vi "RT 4Servos Module.vi"(0 "FPGA VI Reference In":refnum<k20>, 1 "Angle 1":u32=130, 2 "Angle 2":u32=130, 3 "Angle 3":u32=130, 4 "Angle 4":u32=130, 5 "Error In":errorcluster, 6 "Motor 1":enum32{"B", "S", "E", "C"}(ring), 7 "Arm":enum32{"meArm", "uArm"}(ring), 8 "Motor 2":enum32{"B", "S", "E", "C"}(ring)=enum."S", 10 "Motor 3":enum32{"B", "S", "E", "C"}(ring)=enum."E", 11 "No. of Motors":enum32{"1", "2", "3", "4"}(ring), 12 "Motor 4":enum32{"B", "S", "E", "C"}(ring)=enum."C") -> (14 "FPGA VI Reference Out":refnum<k20>, 19 "Error Out":errorcluster)   [LabVIEW 2015]
uses:
  <vilib>/Utility/error.llb/Error Cluster From Error Code.vi
  <vilib>/rvi/errors/niLvFpgaAdjustHostInterfaceError.vi
  <vilib>/rvi/interface/nirviReadWriteControl/nirviReadWriteControl.xnode
  NiFpgaLv.dll
  <vilib>/rvi/interface/Simulation/niFpgaSimulationCallBeginRW.vi
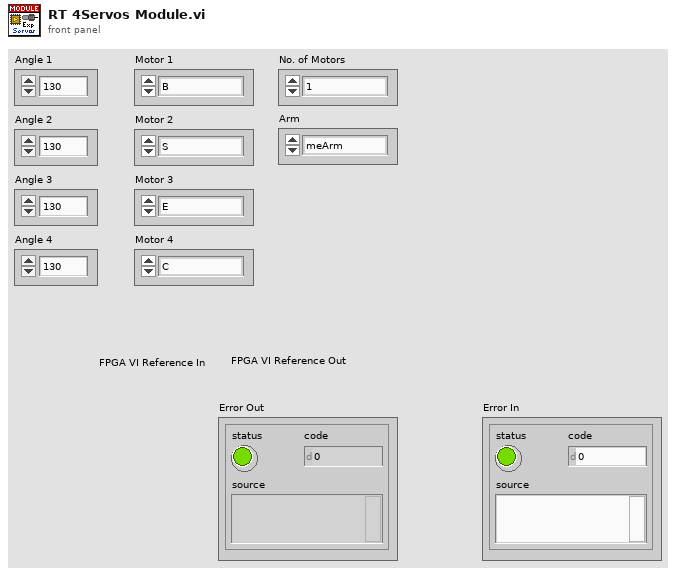
[diagram p1: front panel]
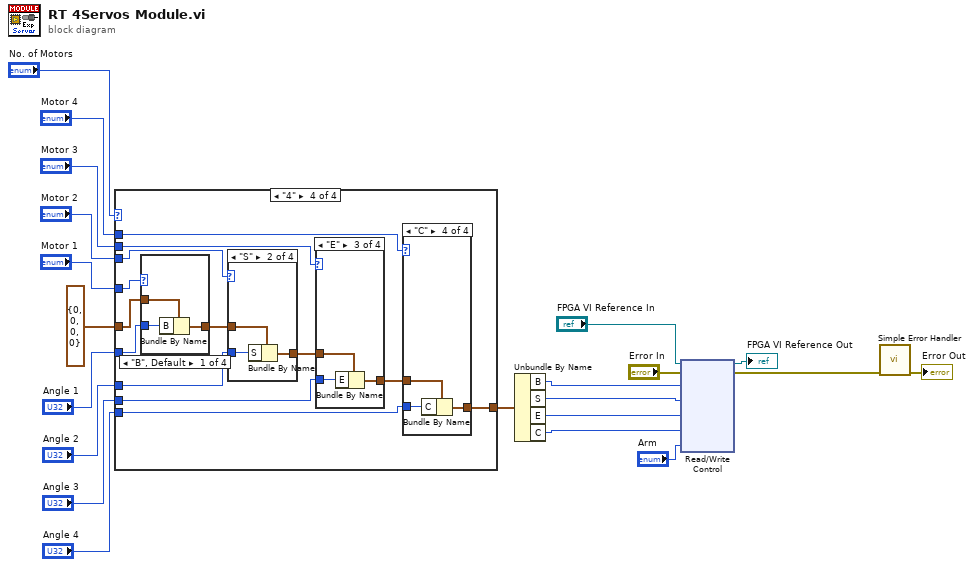
[diagram p0: block diagram]
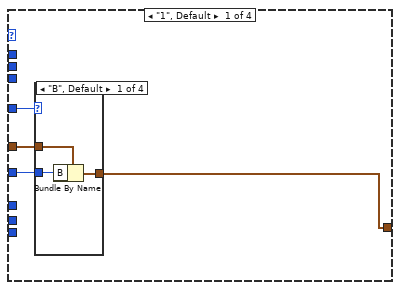
[diagram p2: hidden frame]
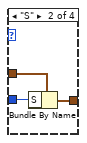
[diagram p3: hidden frame]
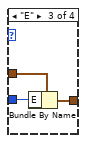
[diagram p4: hidden frame]
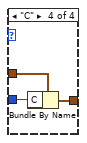
[diagram p5: hidden frame]
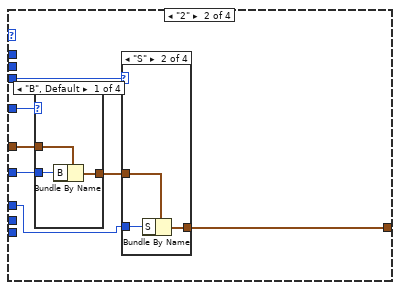
[diagram p6: hidden frame]
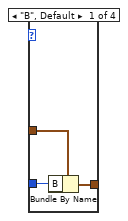
[diagram p7: hidden frame]
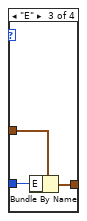
[diagram p8: hidden frame]
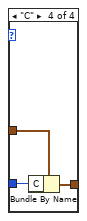
[diagram p9: hidden frame]
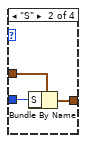
[diagram p10: hidden frame]
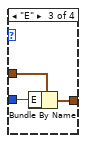
[diagram p11: hidden frame]
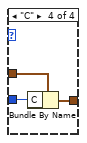
[diagram p12: hidden frame]
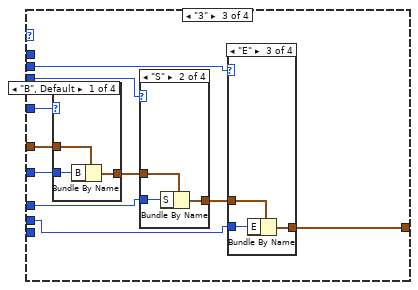
[diagram p13: hidden frame]
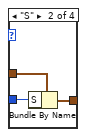
[diagram p14: hidden frame]
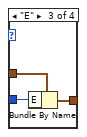
[diagram p15: hidden frame]
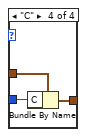
[diagram p16: hidden frame]
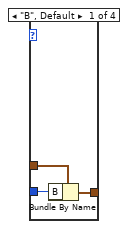
[diagram p17: hidden frame]
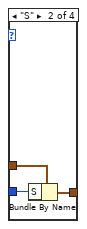
[diagram p18: hidden frame]
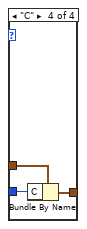
[diagram p19: hidden frame]
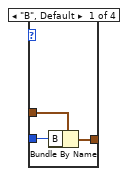
[diagram p20: hidden frame]
diagram:
  n1 = case shown="\"4\"" "No. of Motors" {
    tunnel: "Motor 1" -> [w25 w39 w74 w122]
    tunnel: "Motor 3" -> [_ _ w69 w120]
    tunnel: "Motor 4" -> [_ _ _ w119]
    tunnel: "Motor 2" -> [_ w38 w73 w121]
    tunnel: "Angle 4" -> [_ _ _ w115]
    tunnel: "Angle 2" -> [_ w41 w71 w117]
    tunnel: "Angle 3" -> [_ _ w70 w116]
    tunnel: "Angle 1" -> [w23 w42 w72 w118]
    tunnel: cluster{"B":u32, "S":u32, "E":u32, "C":u32} {"B"=0, "S"=0, "E"=0, "C"=0} ("Servos") -> [w24 w44 w76 w123]
    tunnel: [w22 w43 w77 w124] -> w10
    frame "1", Default {
      n2 = case shown="\"B\", Default" w25 {
        tunnel: w24 -> [w28 w31 w34 w36]
        tunnel: w23 -> [w26 w30 w32 w35]
        tunnel: [w27 w29 w33 w37] -> w22
        frame "B", Default {
          n3 = Bundle By Name(cluster=w28, "B"=w26) -> (w27:cluster{"B":u32, "S":u32, "E":u32, "C":u32})
        }
        frame "S" {
          n4 = Bundle By Name(cluster=w31, "S"=w30) -> (w29:cluster{"B":u32, "S":u32, "E":u32, "C":u32})
        }
        frame "E" {
          n5 = Bundle By Name(cluster=w34, "E"=w32) -> (w33:cluster{"B":u32, "S":u32, "E":u32, "C":u32})
        }
        frame "C" {
          n6 = Bundle By Name(cluster=w36, "C"=w35) -> (w37:cluster{"B":u32, "S":u32, "E":u32, "C":u32})
        }
      }
    }
    frame "2" {
      n7 = case shown="\"B\", Default" w39 {
        tunnel: w44 -> [w59 w62 w65 w68]
        tunnel: w42 -> [w57 w61 w63 w67]
        tunnel: [w58 w60 w64 w66] -> w40
        frame "B", Default {
          n8 = Bundle By Name(cluster=w59, "B"=w57) -> (w58:cluster{"B":u32, "S":u32, "E":u32, "C":u32})
        }
        frame "S" {
          n9 = Bundle By Name(cluster=w62, "S"=w61) -> (w60:cluster{"B":u32, "S":u32, "E":u32, "C":u32})
        }
        frame "E" {
          n10 = Bundle By Name(cluster=w65, "E"=w63) -> (w64:cluster{"B":u32, "S":u32, "E":u32, "C":u32})
        }
        frame "C" {
          n11 = Bundle By Name(cluster=w68, "C"=w67) -> (w66:cluster{"B":u32, "S":u32, "E":u32, "C":u32})
        }
      }
      n12 = case shown="\"S\"" w38 {
        tunnel: w40 -> [w47 w50 w53 w55]
        tunnel: w41 -> [w45 w49 w51 w54]
        tunnel: [w46 w48 w52 w56] -> w43
        frame "B", Default {
          n13 = Bundle By Name(cluster=w47, "B"=w45) -> (w46:cluster{"B":u32, "S":u32, "E":u32, "C":u32})
        }
        frame "S" {
          n14 = Bundle By Name(cluster=w50, "S"=w49) -> (w48:cluster{"B":u32, "S":u32, "E":u32, "C":u32})
        }
        frame "E" {
          n15 = Bundle By Name(cluster=w53, "E"=w51) -> (w52:cluster{"B":u32, "S":u32, "E":u32, "C":u32})
        }
        frame "C" {
          n16 = Bundle By Name(cluster=w55, "C"=w54) -> (w56:cluster{"B":u32, "S":u32, "E":u32, "C":u32})
        }
      }
    }
    frame "3" {
      n17 = case shown="\"B\", Default" w74 {
        tunnel: w76 -> [w81 w84 w87 w90]
        tunnel: w72 -> [w79 w83 w85 w89]
        tunnel: [w80 w82 w86 w88] -> w75
        frame "B", Default {
          n18 = Bundle By Name(cluster=w81, "B"=w79) -> (w80:cluster{"B":u32, "S":u32, "E":u32, "C":u32})
        }
        frame "S" {
          n19 = Bundle By Name(cluster=w84, "S"=w83) -> (w82:cluster{"B":u32, "S":u32, "E":u32, "C":u32})
        }
        frame "E" {
          n20 = Bundle By Name(cluster=w87, "E"=w85) -> (w86:cluster{"B":u32, "S":u32, "E":u32, "C":u32})
        }
        frame "C" {
          n21 = Bundle By Name(cluster=w90, "C"=w89) -> (w88:cluster{"B":u32, "S":u32, "E":u32, "C":u32})
        }
      }
      n22 = case shown="\"S\"" w73 {
        tunnel: w75 -> [w105 w108 w111 w113]
        tunnel: w71 -> [w103 w107 w109 w112]
        tunnel: [w104 w106 w110 w114] -> w78
        frame "B", Default {
          n23 = Bundle By Name(cluster=w105, "B"=w103) -> (w104:cluster{"B":u32, "S":u32, "E":u32, "C":u32})
        }
        frame "S" {
          n24 = Bundle By Name(cluster=w108, "S"=w107) -> (w106:cluster{"B":u32, "S":u32, "E":u32, "C":u32})
        }
        frame "E" {
          n25 = Bundle By Name(cluster=w111, "E"=w109) -> (w110:cluster{"B":u32, "S":u32, "E":u32, "C":u32})
        }
        frame "C" {
          n26 = Bundle By Name(cluster=w113, "C"=w112) -> (w114:cluster{"B":u32, "S":u32, "E":u32, "C":u32})
        }
      }
      n27 = case shown="\"E\"" w69 {
        tunnel: w78 -> [w93 w96 w99 w101]
        tunnel: [w92 w95 w98 w102] -> w77
        tunnel: w70 -> [w91 w94 w97 w100]
        frame "B", Default {
          n28 = Bundle By Name(cluster=w93, "B"=w91) -> (w92:cluster{"B":u32, "S":u32, "E":u32, "C":u32})
        }
        frame "S" {
          n29 = Bundle By Name(cluster=w96, "S"=w94) -> (w95:cluster{"B":u32, "S":u32, "E":u32, "C":u32})
        }
        frame "E" {
          n30 = Bundle By Name(cluster=w99, "E"=w97) -> (w98:cluster{"B":u32, "S":u32, "E":u32, "C":u32})
        }
        frame "C" {
          n31 = Bundle By Name(cluster=w101, "C"=w100) -> (w102:cluster{"B":u32, "S":u32, "E":u32, "C":u32})
        }
      }
    }
    frame "4" {
      n32 = case shown="\"B\", Default" w122 {
        tunnel: w123 -> [w130 w133 w136 w138]
        tunnel: w118 -> [w128 w132 w134 w137]
        tunnel: [w129 w131 w135 w139] -> w127
        frame "B", Default {
          n33 = Bundle By Name(cluster=w130, "B"=w128) -> (w129:cluster{"B":u32, "S":u32, "E":u32, "C":u32})
        }
        frame "S" {
          n34 = Bundle By Name(cluster=w133, "S"=w132) -> (w131:cluster{"B":u32, "S":u32, "E":u32, "C":u32})
        }
        frame "E" {
          n35 = Bundle By Name(cluster=w136, "E"=w134) -> (w135:cluster{"B":u32, "S":u32, "E":u32, "C":u32})
        }
        frame "C" {
          n36 = Bundle By Name(cluster=w138, "C"=w137) -> (w139:cluster{"B":u32, "S":u32, "E":u32, "C":u32})
        }
      }
      n37 = case shown="\"S\"" w121 {
        tunnel: w127 -> [w154 w157 w160 w162]
        tunnel: w117 -> [w152 w156 w158 w161]
        tunnel: [w153 w155 w159 w163] -> w126
        frame "B", Default {
          n38 = Bundle By Name(cluster=w154, "B"=w152) -> (w153:cluster{"B":u32, "S":u32, "E":u32, "C":u32})
        }
        frame "S" {
          n39 = Bundle By Name(cluster=w157, "S"=w156) -> (w155:cluster{"B":u32, "S":u32, "E":u32, "C":u32})
        }
        frame "E" {
          n40 = Bundle By Name(cluster=w160, "E"=w158) -> (w159:cluster{"B":u32, "S":u32, "E":u32, "C":u32})
        }
        frame "C" {
          n41 = Bundle By Name(cluster=w162, "C"=w161) -> (w163:cluster{"B":u32, "S":u32, "E":u32, "C":u32})
        }
      }
      n42 = case shown="\"E\"" w120 {
        tunnel: w126 -> [w166 w169 w172 w174]
        tunnel: w116 -> [w164 w168 w170 w173]
        tunnel: [w165 w167 w171 w175] -> w125
        frame "B", Default {
          n43 = Bundle By Name(cluster=w166, "B"=w164) -> (w165:cluster{"B":u32, "S":u32, "E":u32, "C":u32})
        }
        frame "S" {
          n44 = Bundle By Name(cluster=w169, "S"=w168) -> (w167:cluster{"B":u32, "S":u32, "E":u32, "C":u32})
        }
        frame "E" {
          n45 = Bundle By Name(cluster=w172, "E"=w170) -> (w171:cluster{"B":u32, "S":u32, "E":u32, "C":u32})
        }
        frame "C" {
          n46 = Bundle By Name(cluster=w174, "C"=w173) -> (w175:cluster{"B":u32, "S":u32, "E":u32, "C":u32})
        }
      }
      n47 = case shown="\"C\"" w119 {
        tunnel: w125 -> [w142 w145 w148 w150]
        tunnel: w115 -> [w140 w144 w146 w149]
        tunnel: [w141 w143 w147 w151] -> w124
        frame "B", Default {
          n48 = Bundle By Name(cluster=w142, "B"=w140) -> (w141:cluster{"B":u32, "S":u32, "E":u32, "C":u32})
        }
        frame "S" {
          n49 = Bundle By Name(cluster=w145, "S"=w144) -> (w143:cluster{"B":u32, "S":u32, "E":u32, "C":u32})
        }
        frame "E" {
          n50 = Bundle By Name(cluster=w148, "E"=w146) -> (w147:cluster{"B":u32, "S":u32, "E":u32, "C":u32})
        }
        frame "C" {
          n51 = Bundle By Name(cluster=w150, "C"=w149) -> (w151:cluster{"B":u32, "S":u32, "E":u32, "C":u32})
        }
      }
    }
  }
  n52 = Unbundle By Name(w10) -> ("B"=w4:u32, "S"=w2:u32, "E"=w1:u32, "C"=w3:u32)
  n53 = xnode "Read/Write Control"("FPGA VI Reference In"="FPGA VI Reference In", "error in"="Error In", "S1"=w4, "S2"=w2, "S3"=w1, "S4"=w3, "Arm"="Arm") -> ("FPGA VI Reference Out"=→"FPGA VI Reference Out":refnum<k20>, "error out"=w8:errorcluster)
  n54 = call <vilib>:"Simple Error Handler.vi"("error in (no error)"=w8) -> ("error out"=→"Error Out":errorcluster)  [unwired: 4 in, 4 out]
